vi "WSVCAP SHL Host LL I2C Read.vi"(0 "Bytes to Read":u8=8, 1 "Wait Ticks":u32, 2 "Slave Address":u8, 5 "Sub Address [U8]":u8=191 format="%.0x", 7 "Socket Mask [U64]":u64=1 format="%012x", 11 "error in":errorcluster, 12 "UUT Set (0/1)":u8, 14 "FPGA":T1) -> (4 "C1:1-18 Read Data [DUT Ordered]":u8[][](array[numeric]), 6 "C2:1-18 Read Data [DUT Ordered]":u8[][](array[numeric]), 8 "C3:1-18 Read Data [DUT Ordered]":u8[][](array[numeric]), 10 "Status":u8[](array[numeric]) format="%.0x", 15 "error out":errorcluster)   [LabVIEW 2012]
uses:
  Type Defs/WSVCAP SHL I2C FPGA Enum.ctl
  Type Defs/WSVCAP SHL Top Level Write Read State Enum.ctl
  Type Defs/WSVCAP SHL State.ctl
  Type Defs/WSVCAP SHL Transaction Enum.ctl
  Type Defs/WSVCAP SHL Top Level Control Enum.ctl
  WSVCAP SHL Host LL I2C Debug Global.vi
panel:
  out "Bit Array":u64[](array[numeric]) format="%.0x"
  out "Data Headers":u8[](array[numeric])=[1, 2, 3, 4, 5, 6, 7, 8, 9, 10, 11, 12, 12, 14, 15, 16]
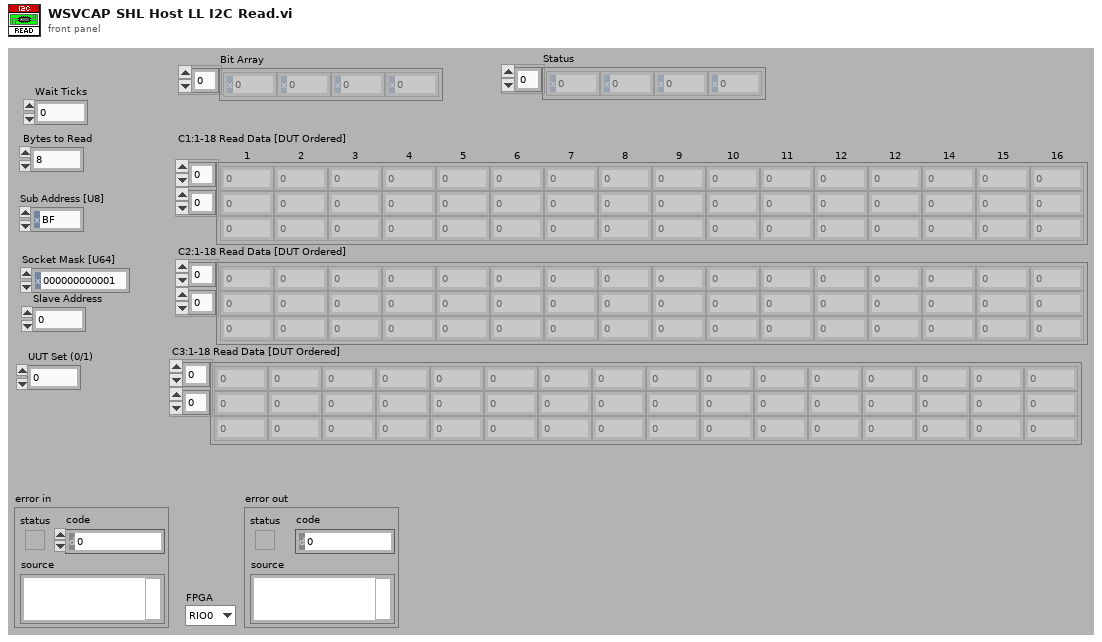
[diagram p1: front panel]
types:
  T1 = typedef "WSVCAP SHL I2C FPGA Enum.ctl" = enum16{"RIO0", "RIO1"}
  T2 = typedef "WSVCAP SHL Top Level Write Read State Enum.ctl" = enum16{"Start", "Write", "Read", "Get Status", "Wait Until Done"}
  T3 = typedef "WSVCAP SHL Transaction Enum.ctl" = enum16{"I2C-Read Data", "I2C-Write Data", "RFFE-Ext Write", "RFFE-Ext Read"}
  T4 = typedef "WSVCAP SHL Top Level Control Enum.ctl" = enum16{"Start", "Cmd", "Transaction", "Wait Ticks", "Socket Mask", "UUT Set", "Slave Address", "Sub Address", "Bytes to Write", "Bytes to Read", "Write Data", "Write Flag", "Read Data", "Read Flag", "Ack Read", "Read Status Flag", "Ack Read Status", "Status", "Cycle Count", "Stop Cycle", "Exit"}
  T5 = typedef "WSVCAP SHL State.ctl" = enum8{"Idle", "Transfer Data"}
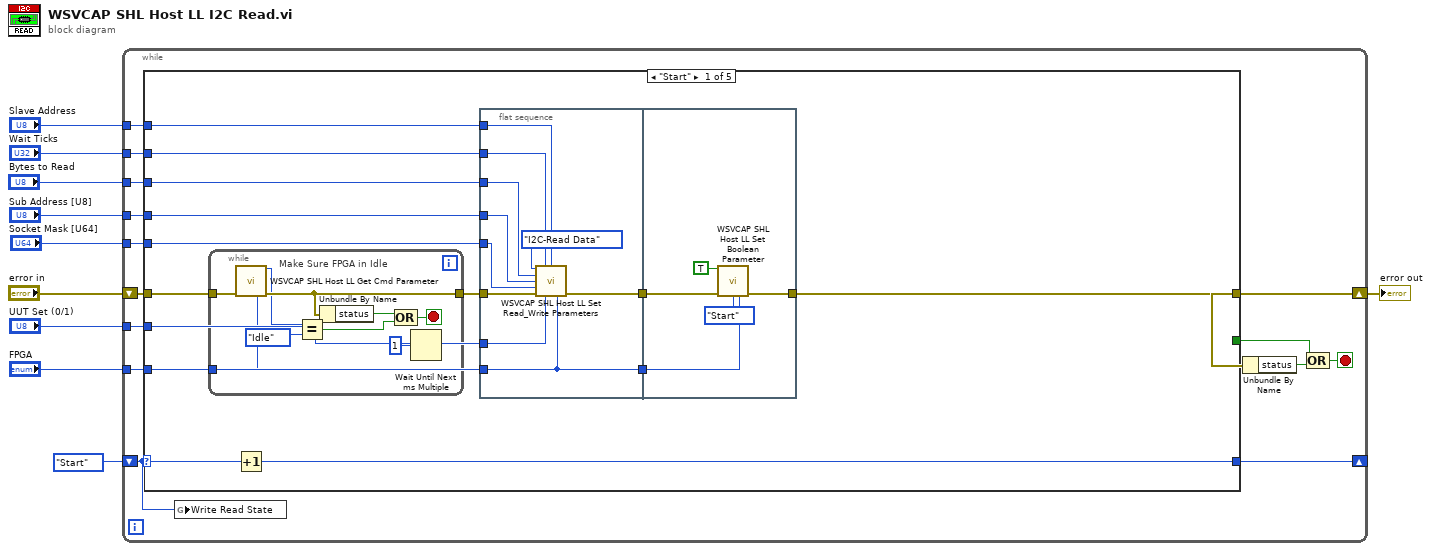
[diagram p0: block diagram]
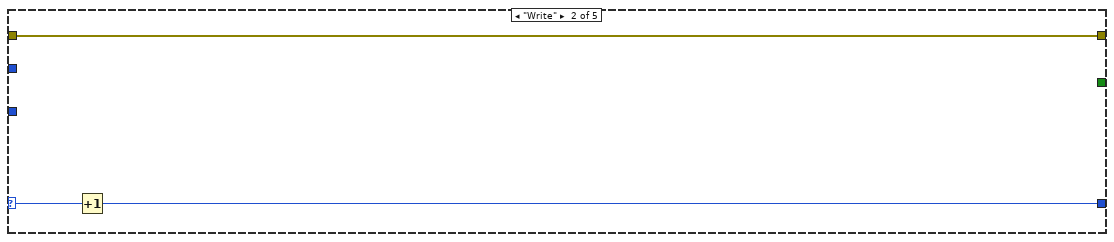
[diagram p2: hidden frame]
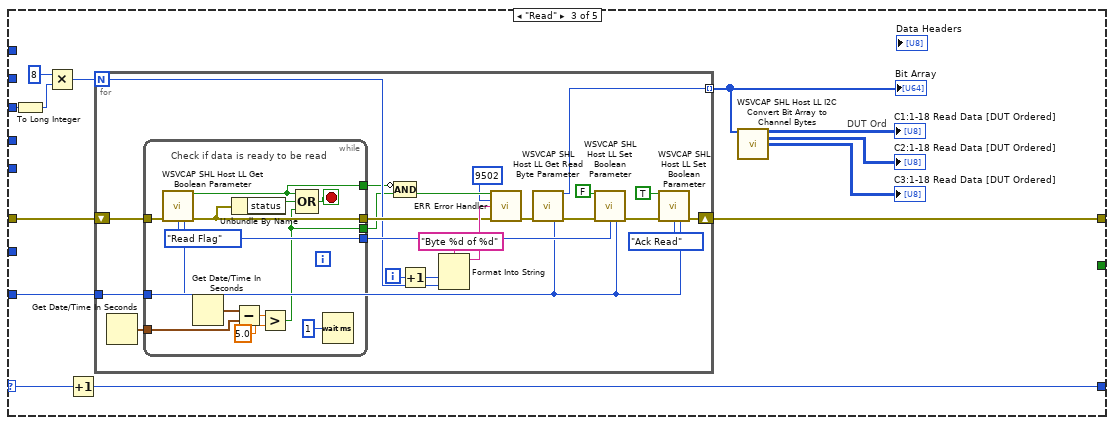
[diagram p3: hidden frame]
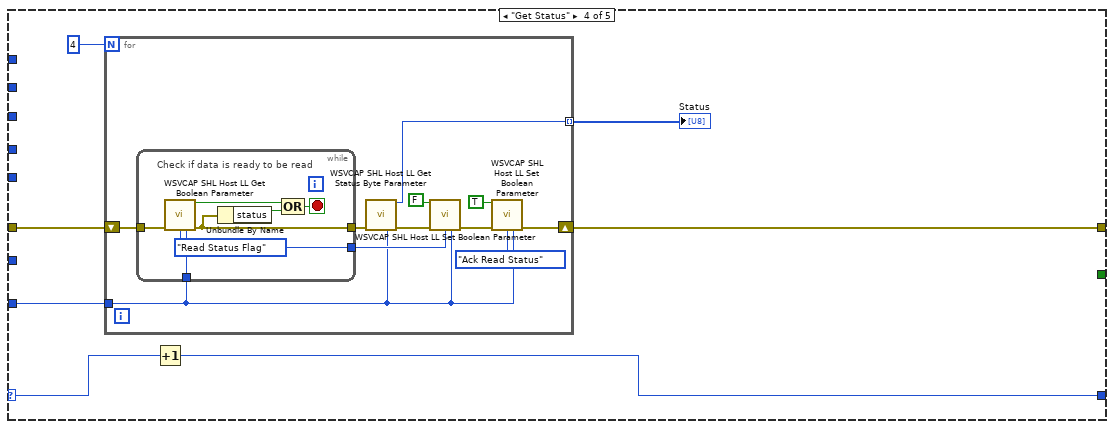
[diagram p4: hidden frame]
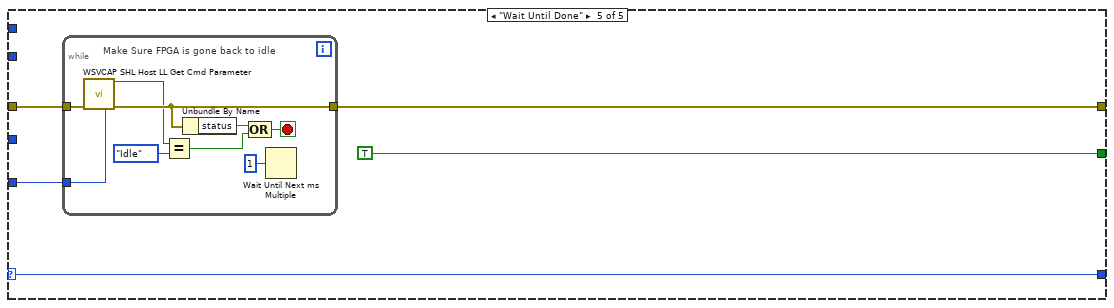
[diagram p5: hidden frame]
diagram:
  n1 = while {
    shift-right: [w23] -> w9
    shift-left: "error in" -> [w24]
    shift-right: [w19] -> _
    shift-left: WSVCAP_SHL_Top_Level_Write_Read_State_Enum."Start" ("Write Read State") -> [w11]
    tunnel: "Bytes to Read" -> [w18]
    tunnel: "Sub Address [U8]" -> [w17]
    tunnel: "Socket Mask [U64]" -> [w16]
    tunnel: "Wait Ticks" -> [w15]
    tunnel: "Slave Address" -> [w14]
    tunnel: "UUT Set (0/1)" -> [w13]
    tunnel: "FPGA" -> [w12]
    stop <- w20 stop-if-true
    n2 = case shown="\"Start\"" w11 {
      selector: w11 -> [w37 w63 w76 w117 w140]
      tunnel: w24 -> [w38 w62 w69 w119 w142]
      tunnel: [w33 w62 w77 w118 w141] -> w23
      tunnel: [_ _ _ _ TRUE] -> w22
      tunnel: [w36 w64 w75 w116 w140] -> w19
      tunnel: w18 -> [w35 _ w74 _ _]
      tunnel: w17 -> [w31 _ _ _ _]
      tunnel: w16 -> [w30 _ _ _ _]
      tunnel: w15 -> [w29 _ _ _ _]
      tunnel: w14 -> [w28 _ _ _ _]
      tunnel: w13 -> [w27 _ _ _ _]
      tunnel: w12 -> [w26 _ w65 w113 w138]
      frame "Start" {
        n3 = while {
          tunnel: w38 -> [w57]
          tunnel: [w56] -> w34
          tunnel: w26 -> [w53]
          stop <- w61 stop-if-true
          # "Make Sure FPGA in Idle"
          n4 = call "WSVCAP SHL Host LL Get Cmd Parameter.vi"("error in (no error)"=w57, "FPGA"=w53) -> ("I2C_Cmd"=w55:T5, "error out"=w56:errorcluster)  [unwired: 12 in]
          n5 = Equal?(x=w55, y=WSVCAP_SHL_State."Idle" ("Type")) -> (x = y?=w59:bool)
          n6 = Unbundle By Name(w56) -> ("status"=w54:bool)
          n7 = Compound Arithmetic op=OR(w54, w59) -> (w61:bool)
          n8 = Wait Until Next ms Multiple(millisecond multiple=u32 1) -> ()  [unwired: 1 out]
        }
        n9 = Increment(x=w37) -> (x+1=w36:T2)
        n10 = flat-sequence {
          tunnel: w35 -> [w45]
          tunnel: w34 -> [w48]
          tunnel: [w46] -> w32
          tunnel: w31 -> [w43]
          tunnel: w30 -> [w44]
          tunnel: w29 -> [w42]
          tunnel: w28 -> [w41]
          tunnel: w27 -> [w40]
          tunnel: w26 -> [w39]
          tunnel: [w39] -> w25
          tunnel: [w52] -> w33
          tunnel: w32 -> [w52]
          tunnel: w25 -> [w49]
          frame #0 {
            n11 = call "WSVCAP SHL Host LL Set Read_Write Parameters.vi"("Transaction"=WSVCAP_SHL_Transaction_Enum."I2C-Read Data", "Wait Ticks"=w42, "Slave Address"=w41, "Bytes"=w45, "Sub Address [U8]"=w43, "Socket Mask [U64]"=w44, "error in (no error)"=w48, "UUT Set (0/1)"=w40, "FPGA"=w39) -> ("error out"=w46:errorcluster)  [unwired: 6 in]
          }
          frame #1 {
            n12 = call "WSVCAP SHL Host LL Set Boolean Parameter.vi"("Boolean In"=TRUE, "error in (no error)"=w52, "FPGA Top Level Control"=WSVCAP_SHL_Top_Level_Control_Enum."Start", "FPGA"=w49) -> ()  [unwired: 11 in, 1 out]
          }
        }
      }
      frame "Write" {
        n13 = Increment(x=w63) -> (x+1=w64:T2)
      }
      frame "Read" {
        # "DUT Ord"
        n14 = To Long Integer(number=w74) -> (32bit integer=w73:i32)
        n15 = Multiply(x=8, y=w73) -> (x*y=w71:i32)
        n16 = Increment(x=w76) -> (x+1=w75:T2)
        n17 = for {
          N: w71 -> [w82]
          shift-right: [w97] -> w77
          shift-left: w69 -> [w99]
          tunnel: [w91] -> w72 mode=indexing
          tunnel: w65 -> [w78]
          i -> [w83]
          n18 = Get Date/Time In Seconds() -> (seconds since 1Jan1904=w79:timestamp)
          n19 = while {
            tunnel: w99 -> [w111]
            tunnel: [w110] -> w85
            tunnel: [w108] -> w96
            tunnel: w79 -> [w105]
            tunnel: [w102] -> w81
            tunnel: [w101] -> w80
            tunnel: w78 -> [w100]
            stop <- w112 stop-if-true
            w108 = WSVCAP_SHL_Top_Level_Control_Enum."Read Flag" ("FPGA Top Level Control")
            # "Check if data is ready to be read"
            n20 = call "WSVCAP SHL Host LL Get Boolean Parameter.vi"("error in (no error)"=w111, "FPGA Top Level Control"=w108, "FPGA"=w100) -> ("Boolean Out"=w102:bool, "error out"=w110:errorcluster)  [unwired: 11 in]
            n21 = Get Date/Time In Seconds() -> (seconds since 1Jan1904=w106:timestamp)
            n22 = Unbundle By Name(w110) -> ("status"=w109:bool)
            n23 = Subtract(x=w106, y=w105) -> (x-y=w104:dbl)
            n24 = Greater?(x=w104, y=5.0) -> (0:w101:bool)
            n25 = Compound Arithmetic op=OR(w102, w109, w101) -> (w112:bool)
            n26 = Wait (ms)(milliseconds to wait=u32 1) -> ()  [unwired: 1 out]
          }
          n27 = Compound Arithmetic op=AND(invert w81, w80) -> (w90:bool)
          n28 = Increment(x=w83) -> (x+1=w86:i32)
          n29 = Format Into String(format string="Byte %d of %d", w86, w82) -> (resulting string=w88:string)  [unwired: 2 in, 1 out]
          n30 = call "ERR Error Handler.vi"("Error Status"=w90, "Error Code"=9502, "Cause Of Error"=w88, "Error In (no error)"=w85) -> ("Error Out"=w84:errorcluster)  [unwired: 11 in]
          n31 = call "WSVCAP SHL Host LL Get Read Byte Parameter.vi"("error in (no error)"=w84, "FPGA"=w78) -> ("Read Data In"=w91:u64, "error out"=w98:errorcluster)  [unwired: 12 in]
          n32 = call "WSVCAP SHL Host LL Set Boolean Parameter.vi"("Boolean In"=FALSE ("Read Flag"), "error in (no error)"=w98, "FPGA Top Level Control"=w96, "FPGA"=w78) -> ("error out"=w92:errorcluster)  [unwired: 11 in]
          n33 = call "WSVCAP SHL Host LL Set Boolean Parameter.vi"("Boolean In"=TRUE ("Write Flag"), "error in (no error)"=w92, "FPGA Top Level Control"=WSVCAP_SHL_Top_Level_Control_Enum."Ack Read", "FPGA"=w78) -> ("error out"=w97:errorcluster)  [unwired: 11 in]
        }
        "Bit Array" <- w72
        n34 = call "WSVCAP SHL Host LL I2C Convert Bit Array to Channel Bytes.vi"("Bit Array"=w72) -> ("C1:1-18 Read Data [SKT Ordered]"=→"C1:1-18 Read Data [DUT Ordered]":u8[][], "C2:1-18 Read Data [SKT Ordered]"=→"C2:1-18 Read Data [DUT Ordered]":u8[][], "C3:1-18 Read Data [SKT Ordered]"=→"C3:1-18 Read Data [DUT Ordered]":u8[][])  [unwired: 12 in]
      }
      frame "Get Status" {
        n35 = for {
          N: 4 -> [_]
          shift-right: [w127] -> w118
          shift-left: w119 -> [w130]
          tunnel: [w121] -> w115 mode=indexing
          tunnel: w113 -> [w120]
          n36 = while {
            tunnel: w130 -> [w135]
            tunnel: [w134] -> w129
            tunnel: [w132] -> w126
            tunnel: w120 -> [w131]
            stop <- w137 stop-if-true
            w132 = WSVCAP_SHL_Top_Level_Control_Enum."Read Status Flag" ("FPGA Top Level Control")
            # "Check if data is ready to be read"
            n37 = call "WSVCAP SHL Host LL Get Boolean Parameter.vi"("error in (no error)"=w135, "FPGA Top Level Control"=w132, "FPGA"=w131) -> ("Boolean Out"=w136:bool, "error out"=w134:errorcluster)  [unwired: 11 in]
            n38 = Unbundle By Name(w134) -> ("status"=w133:bool)
            n39 = Compound Arithmetic op=OR(w136, w133) -> (w137:bool)
          }
          n40 = call "WSVCAP SHL Host LL Get Status Byte Parameter.vi"("error in (no error)"=w129, "FPGA"=w120) -> ("I2C Status Byte"=w121:u8, "error out"=w128:errorcluster)  [unwired: 12 in]
          n41 = call "WSVCAP SHL Host LL Set Boolean Parameter.vi"("Boolean In"=FALSE ("Read Flag"), "error in (no error)"=w128, "FPGA Top Level Control"=w126, "FPGA"=w120) -> ("error out"=w122:errorcluster)  [unwired: 11 in]
          n42 = call "WSVCAP SHL Host LL Set Boolean Parameter.vi"("Boolean In"=TRUE ("Write Flag"), "error in (no error)"=w122, "FPGA Top Level Control"=WSVCAP_SHL_Top_Level_Control_Enum."Ack Read Status", "FPGA"=w120) -> ("error out"=w127:errorcluster)  [unwired: 11 in]
        }
        "Status" <- w115
        n43 = Increment(x=w117) -> (x+1=w116:T2)
      }
      frame "Wait Until Done" {
        n44 = while {
          tunnel: w142 -> [w146]
          tunnel: [w145] -> w141
          tunnel: w138 -> [w143]
          stop <- w148 stop-if-true
          # "Make Sure FPGA is gone back to idle"
          n45 = call "WSVCAP SHL Host LL Get Cmd Parameter.vi"("error in (no error)"=w146, "FPGA"=w143) -> ("I2C_Cmd"=w144:T5, "error out"=w145:errorcluster)  [unwired: 12 in]
          n46 = Equal?(x=w144, y=WSVCAP_SHL_State."Idle") -> (x = y?=w149:bool)
          n47 = Unbundle By Name(w145) -> ("status"=w150:bool)
          n48 = Compound Arithmetic op=OR(w150, w149) -> (w148:bool)
          n49 = Wait Until Next ms Multiple(millisecond multiple=u32 1) -> ()  [unwired: 1 out]
        }
      }
    }
    n50 = global write "WSVCAP SHL Host LL I2C Debug Global.vi" "Write Read State"(w11) -> ()
    n51 = Unbundle By Name(w23) -> ("status"=w21:bool)
    n52 = Compound Arithmetic op=OR(w22, w21) -> (w20:bool)
  }
  "error out" <- w9
